vi "Snap (Express).vi"() -> ()   [LabVIEW 2011]
doc: "The Snap (Express) VI acquires an image and displays the image in an image control using the Vision Acquisition Express VI. A snap is appropriate for single-capture applications in which ease of programming is essential."
uses:
  Instance           2 22Saved   Snap (Express) .vi
panel:
  out "Image":T1(plugin-control)
  # "Overview: Demonstrates how to acquire a single image.\nRequirements: Vision Acquisition Software\nInstructions: Run the VI"
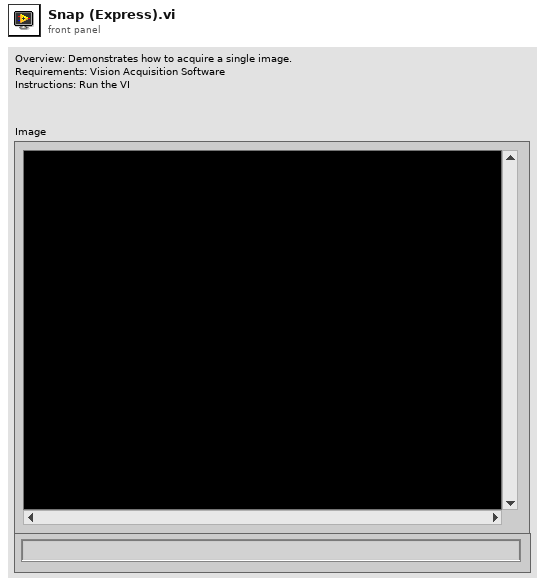
[diagram p1: front panel]
types:
  T1 = typedef "IMAQ Image.ctl" = refnum<image>
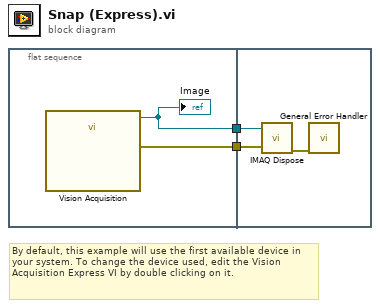
[diagram p0: block diagram]
diagram:
  # "By default, this example will use the first available device in your system. To change the device used, edit the Vision Acquisition Express VI by double clicking on it."
  n1 = flat-sequence {
    tunnel: [w4] -> w2
    tunnel: [w3] -> w1
    tunnel: w2 -> [w7]
    tunnel: w1 -> [w6]
    frame #0 {
      n2 = call "Vision Acquisition"() -> ("Image Out"=w4:T1, "error out"=w3:errorcluster)  [unwired: 1 in, 25 out]
      "Image" <- w4
    }
    frame #1 {
      n3 = call "IMAQ Dispose"("Image"=w7, "error in (no error)"=w6) -> ("error out"=w5:errorcluster)  [unwired: 4 in]
      n4 = call <vilib>:"General Error Handler.vi"("error in (no error)"=w5) -> ()  [unwired: 1 in, 14 out]
    }
  }
